vi "global.vi"() -> ()   [LabVIEW 2011]
panel:
  out "Events":dbl[][](array[numeric])
  in  "Path to recived data from motes":path=path "C:/HVAC/log/motes.txt"
  in  "path to occupancy":path=path "C:/Users/HVACProject/Dropbox/HVACProject/Website/HVAC/Graph/occupancy.jpeg"
  in  "path to co2":path=path "C:/Users/HVACProject/Dropbox/HVACProject/Website/HVAC/Graph/co2.jpeg"
  in  "path to humidity":path=path "C:/Users/HVACProject/Dropbox/HVACProject/Website/HVAC/Graph/humi.jpeg"
  in  "path to temp":path=path "C:/Users/HVACProject/Dropbox/HVACProject/Website/HVAC/Graph/temp.jpeg"
  in  "database backup PATH (remote PC)":string="\\\\BACKUPUSER-PC\\backup_PC"
  out "+4 Day Hourly Forecast":string[][](array[string])
  out "+3 Day Hourly Forecast":string[][](array[string])
  out "+2 Day Hourly Forecast":string[][](array[string])
  out "+1 Day Hourly Forecast":string[][](array[string])
  out "Now":string[][](array[string])
  out "Today Hourly Forecast":string[][](array[string])
  in  "database backup PATH (local PC)":string="C:\\HVAC\\database_backup"
  in  "database PATH":string="C:\\HVAC\\database\\mydatabase.sqlite"
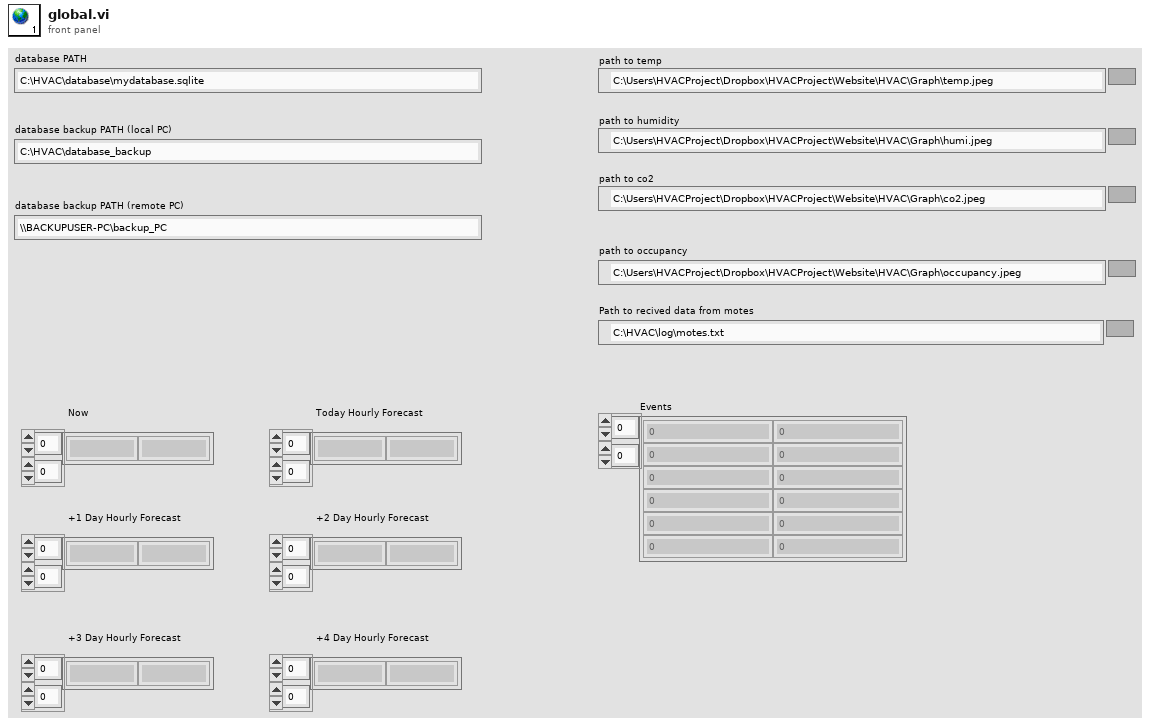
[diagram p1: front panel]
diagram:
